vi "LC-MISDK_UserCalibration__.vi"() -> ()   [LabVIEW 2015]
uses:
  C:/Program Files (x86)/National Instruments/LabVIEW 2015/LC-MISDK.dll
  Program Files (x86)/National Instruments/LabVIEW 2015/LC-MISDK.dll
panel:
  in  "タイムスタンプ":timestamp
  out "数値":dbl
  out "error out":errorcluster caption="エラー出力"
  out "ErrorCode":dbl
  in  "Before_B 2":bool
  in  "Before_G 2":bool
  in  "Before_R 2":bool
  in  "Before_W 2":bool
  in  "After_B":T1
  in  "After_G":T2
  in  "After_R":T3
  in  "After_W":T4
  in  "Before_B":T5
  in  "Before_G":T6
  in  "Before_R":T7
  in  "Before_W":T8
  out "Error Message":string
  in  "EXIT":bool
  in  "Calib":bool
  in  "ID":string
  in  "Color Space":T9(ring)
  in  "Calib.Ch":T10(ring)
  in  "Type of Calibration":enum32{"Single-Point", "RGB", "WRGB"}(radio)
  # "Value before Calibration"
  # "Value after Calibration"
  # "Lv"
  # "u"
  # "v"
  # "Lv"
  # "u"
  # "v"
  # "White"
  # "White"
  # "Red"
  # "Red"
  # "Green"
  # "Green"
  # "Blue"
  # "Blue"
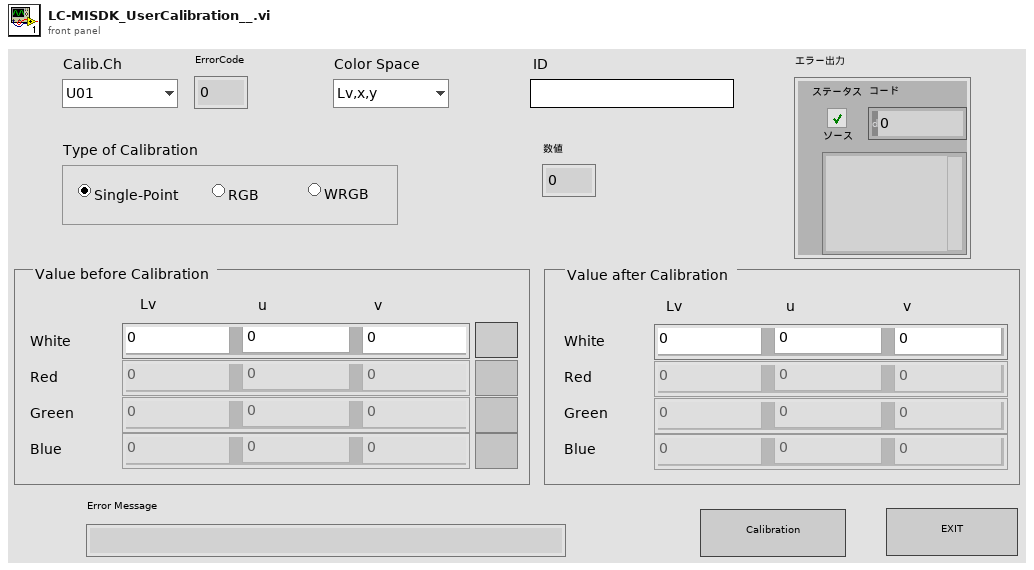
[diagram p1: front panel]
types:
  T1 = cluster{"After_B1":dbl, "After_B2":dbl, "After_B3":dbl}
  T2 = cluster{"After_G1":dbl, "After_G2":dbl, "After_G3":dbl}
  T3 = cluster{"After_R1":dbl, "After_R2":dbl, "After_R3":dbl}
  T4 = cluster{"After_W1":dbl, "After_W2":dbl, "After_W3":dbl}
  T5 = cluster{"before_B1":dbl, "Before_B2":dbl, "Before_B3":dbl}
  T6 = cluster{"before_G1":dbl, "Before_G2":dbl, "Before_G3":dbl}
  T7 = cluster{"before_R1":dbl, "Before_R2":dbl, "Before_R3":dbl}
  T8 = cluster{"before_W1":dbl, "Before_W2":dbl, "Before_W3":dbl}
  T9 = enum16{"Lv,x,y", "Lv,u',v'", "Lv,Tcp,duv", "X,Y,Z", "Lv,λd,Pe"}
  T10 = enum16{"U01", "U02", "U03", "U04", "U05", "U06", "U07", "U08", "U09", "U10"}
  T11 = cluster{"get_Item":dbl, "get_Item":dbl, "get_Item":dbl}
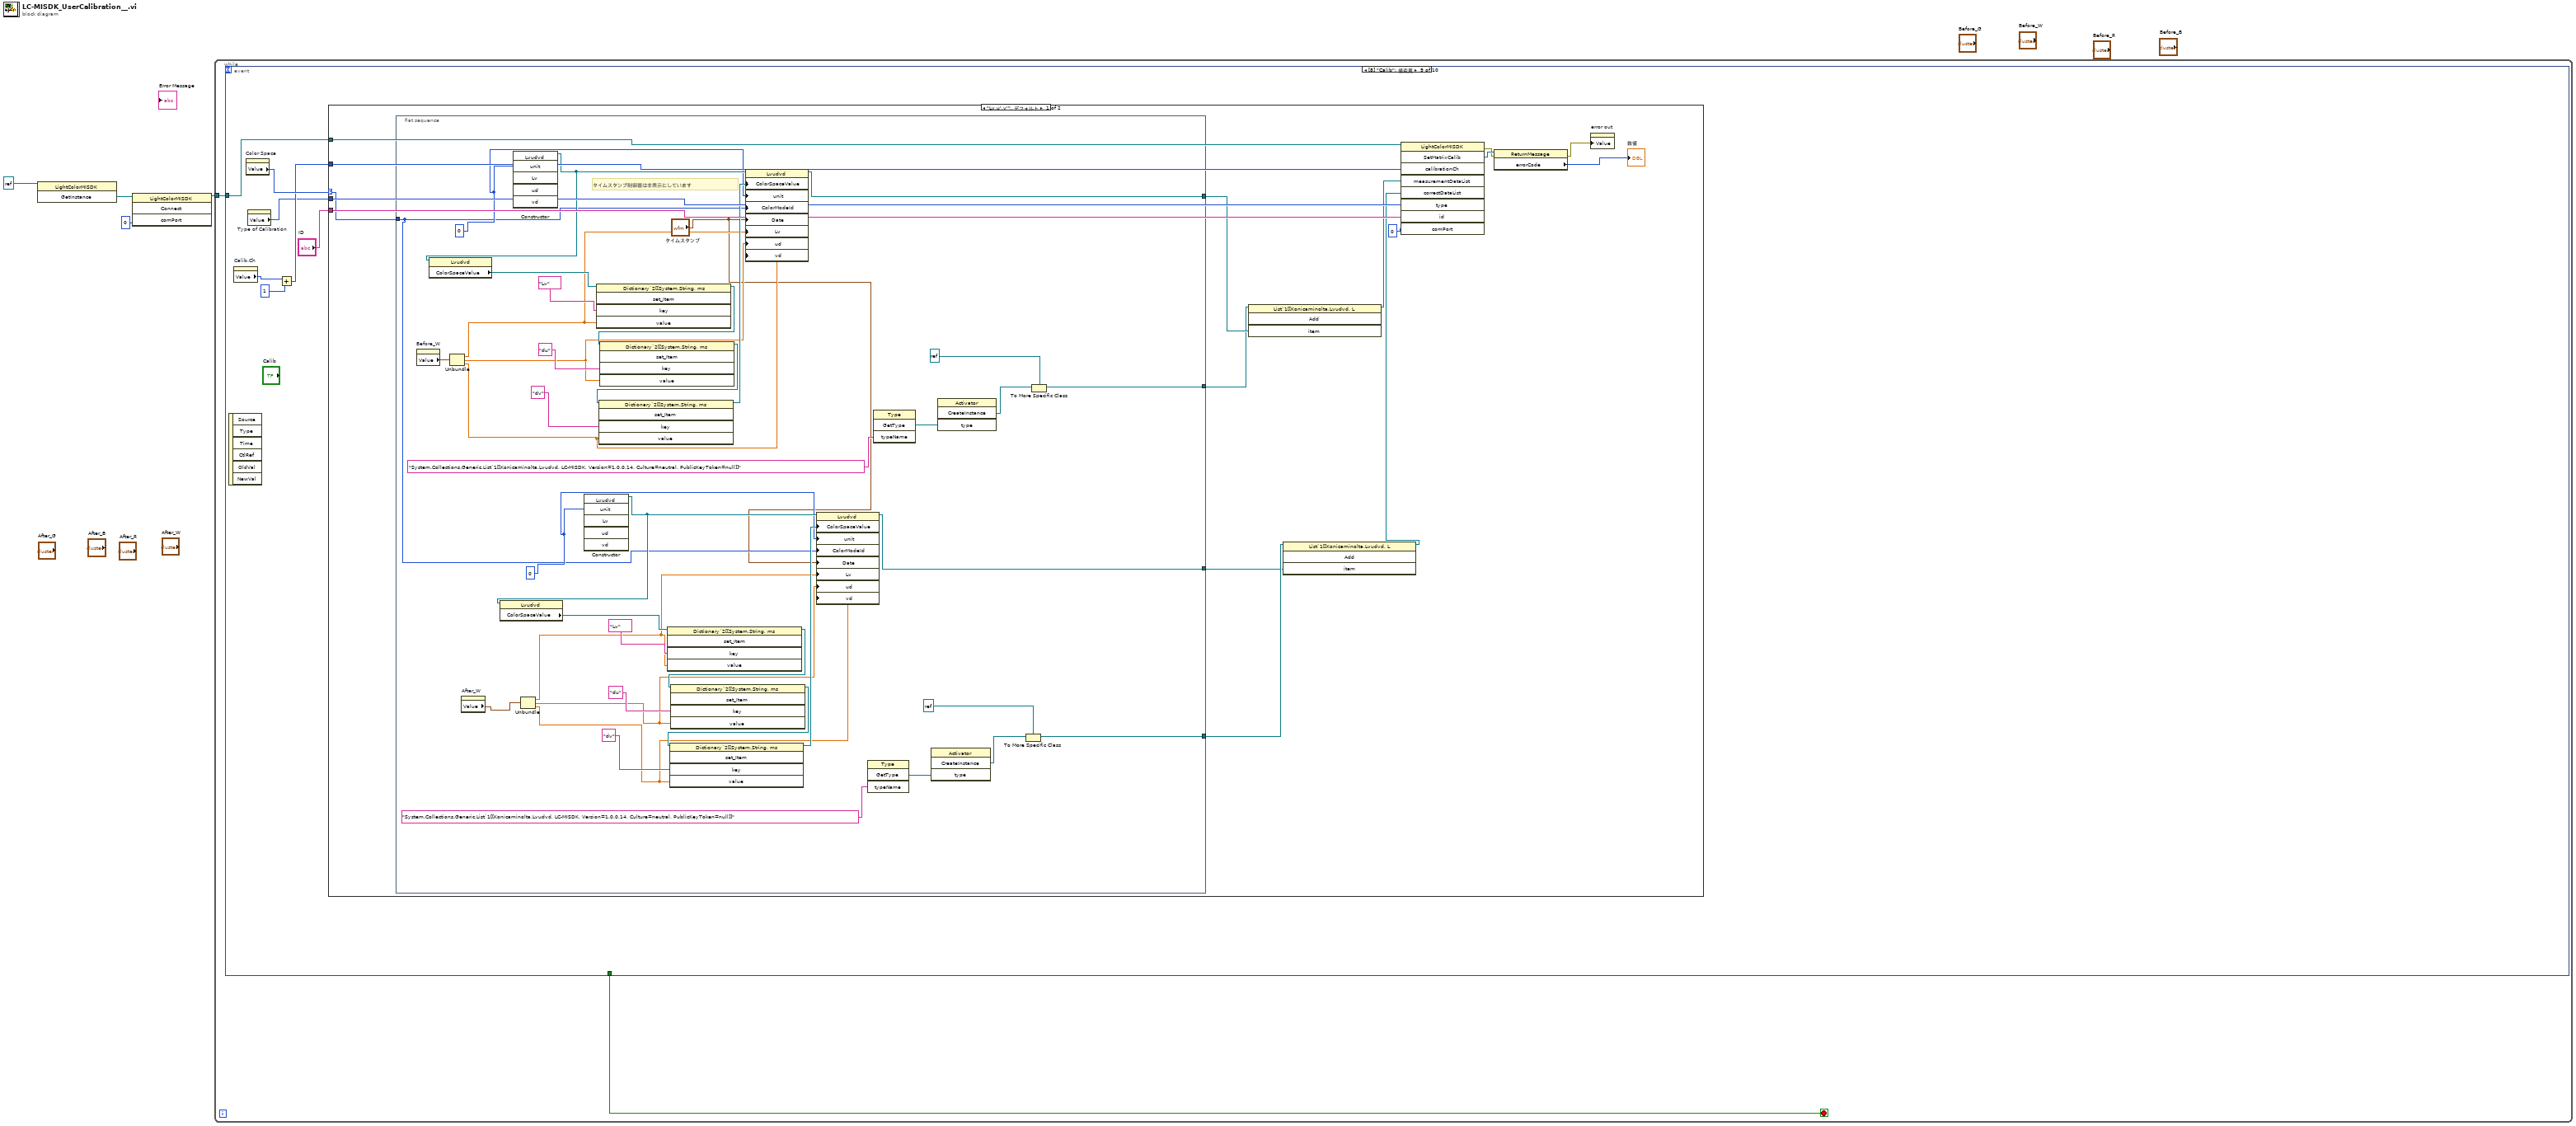
[diagram p0: block diagram]
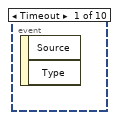
[diagram p2: hidden frame]
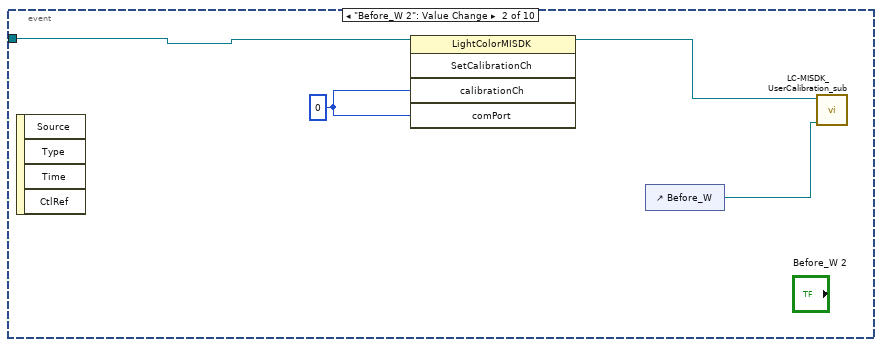
[diagram p3: hidden frame]
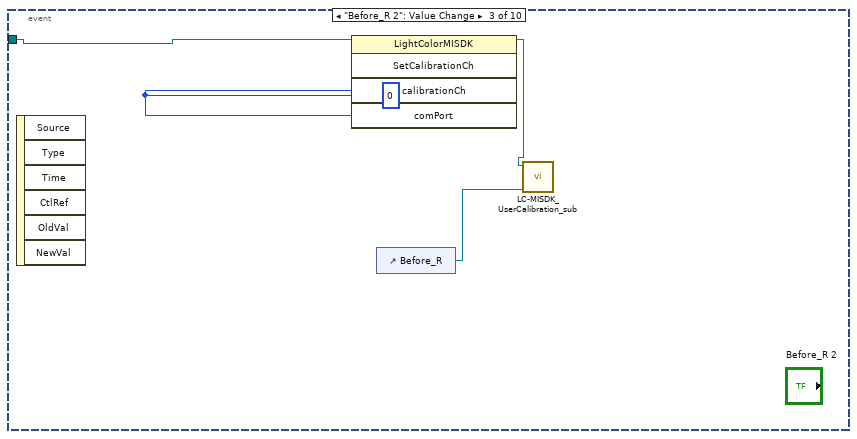
[diagram p4: hidden frame]
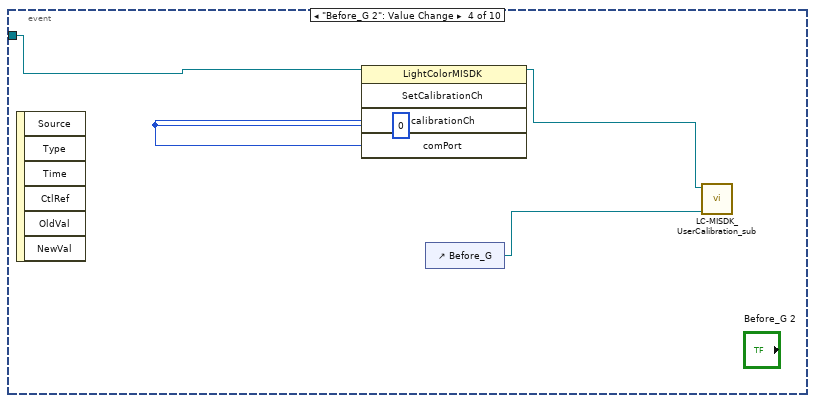
[diagram p5: hidden frame]
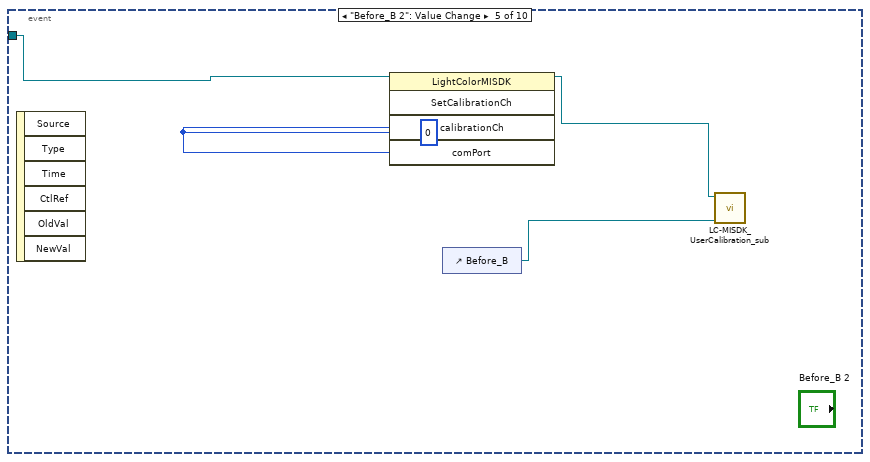
[diagram p6: hidden frame]
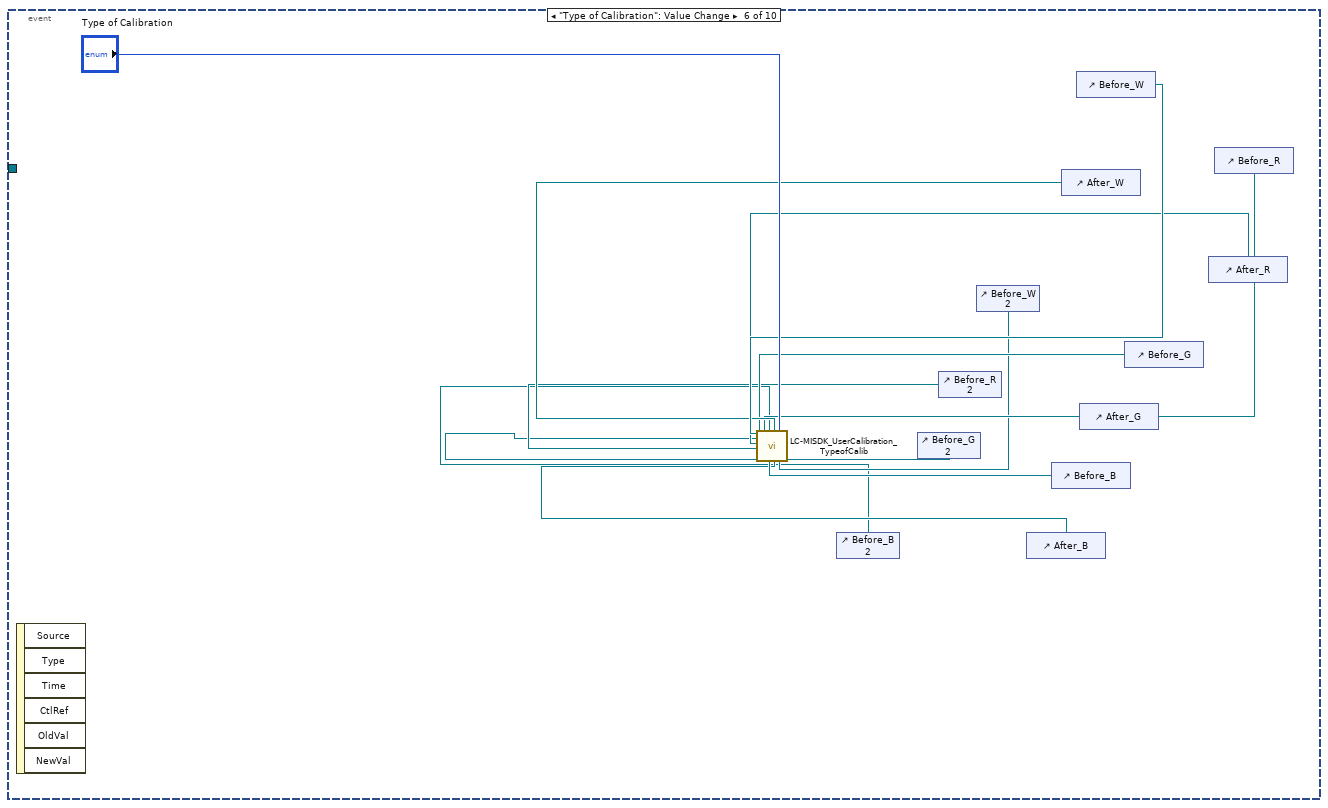
[diagram p7: hidden frame]
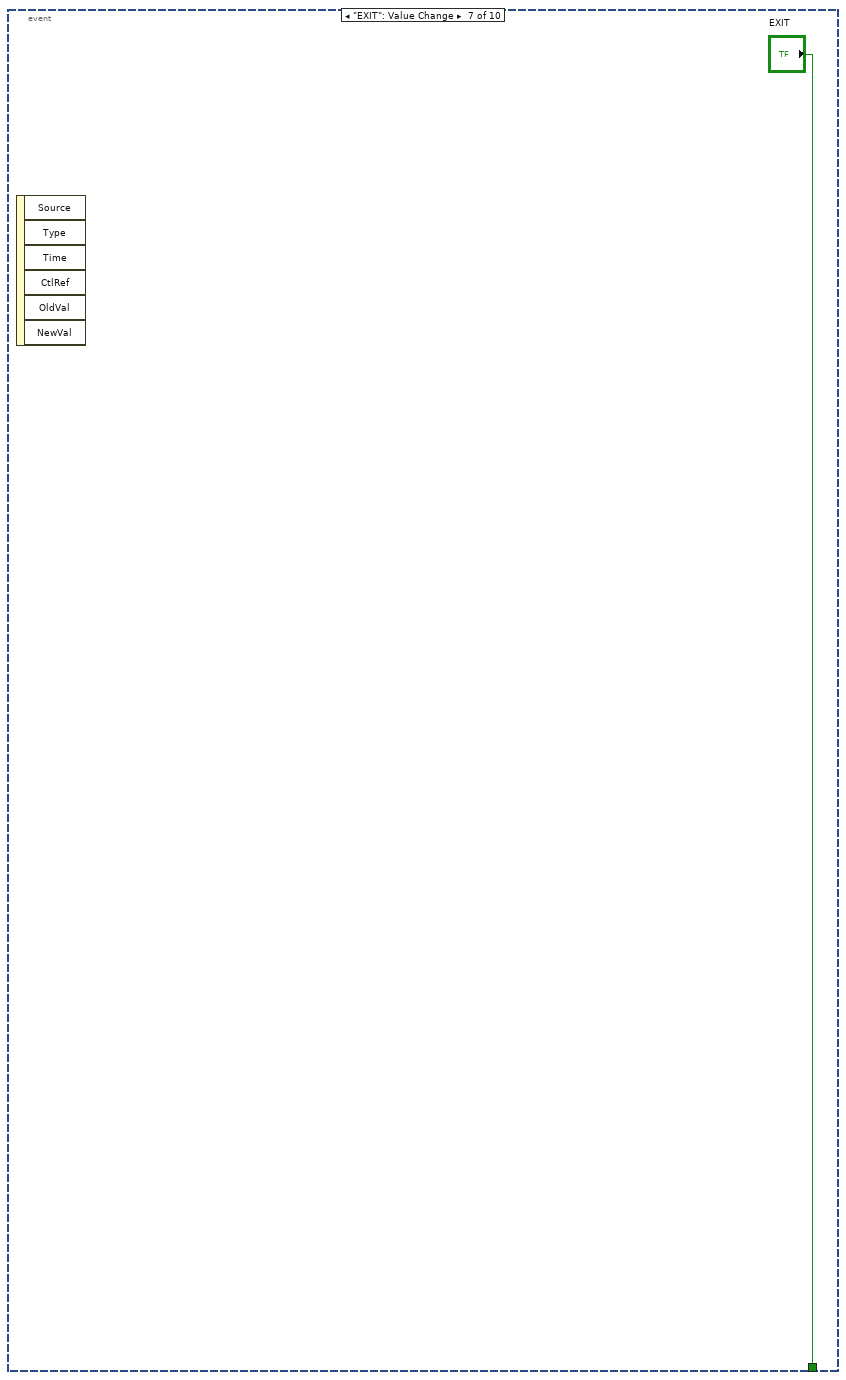
[diagram p8: hidden frame]
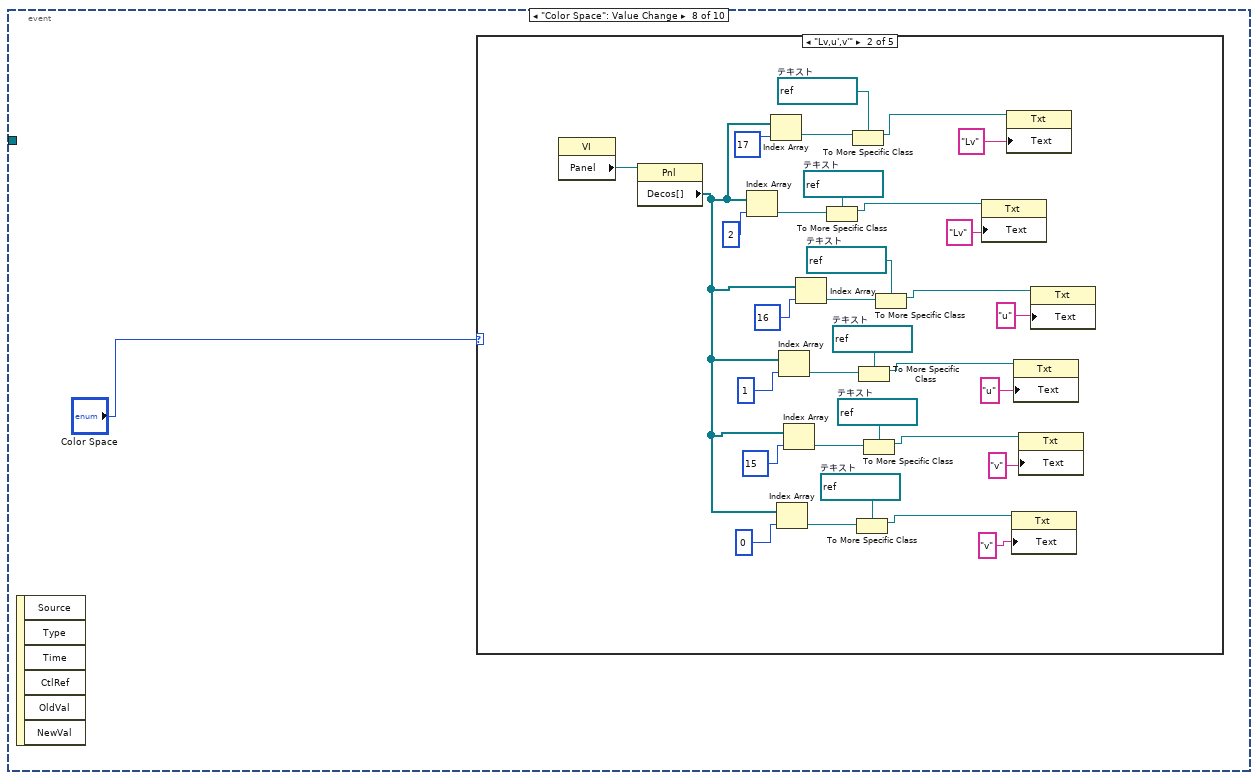
[diagram p9: hidden frame]
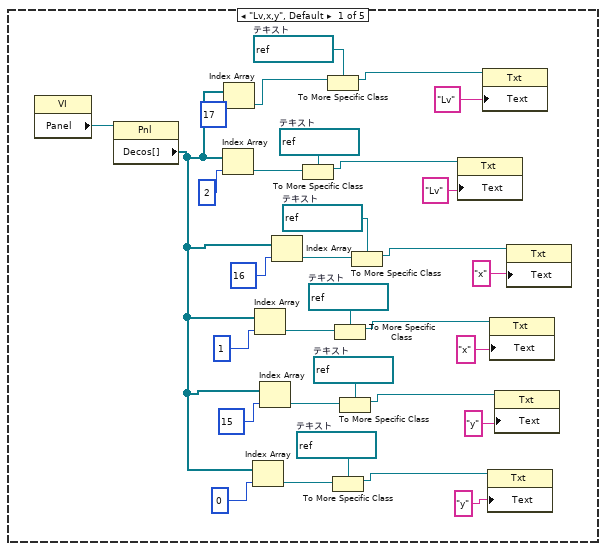
[diagram p10: hidden frame]
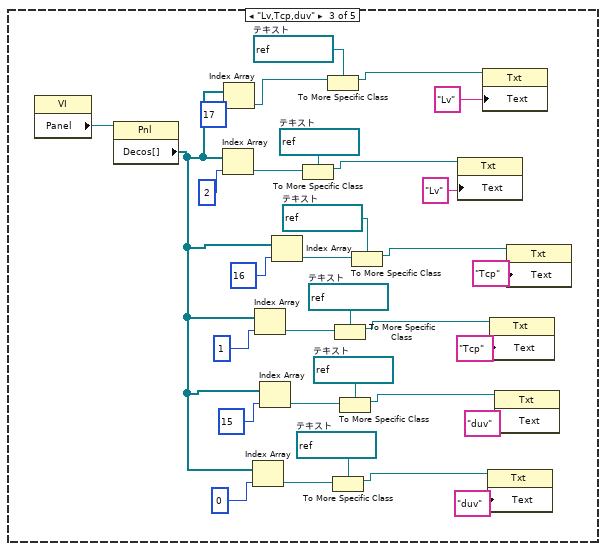
[diagram p11: hidden frame]
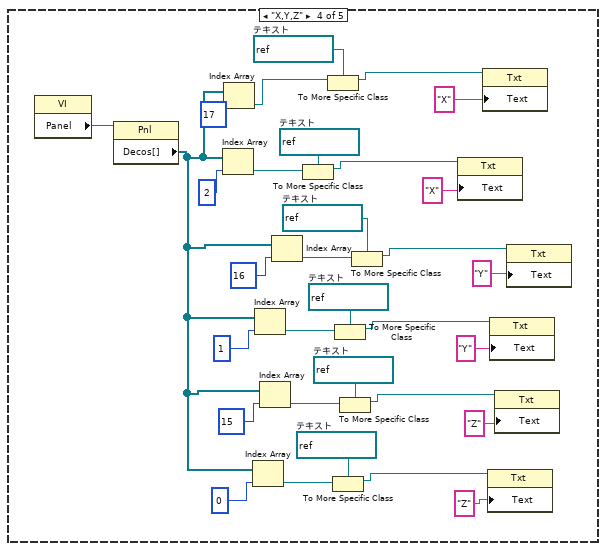
[diagram p12: hidden frame]
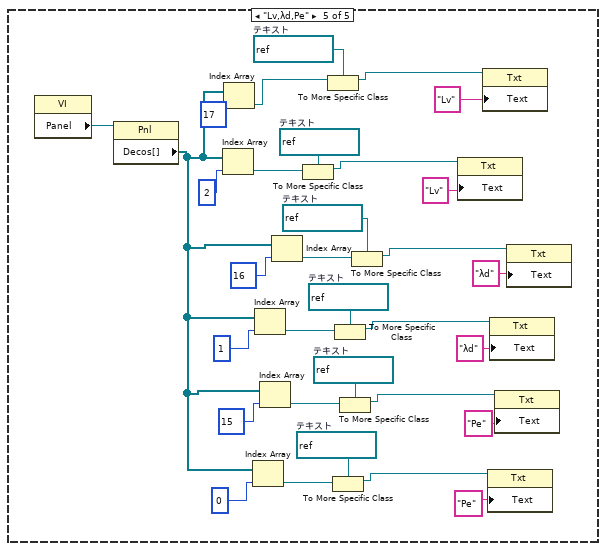
[diagram p13: hidden frame]
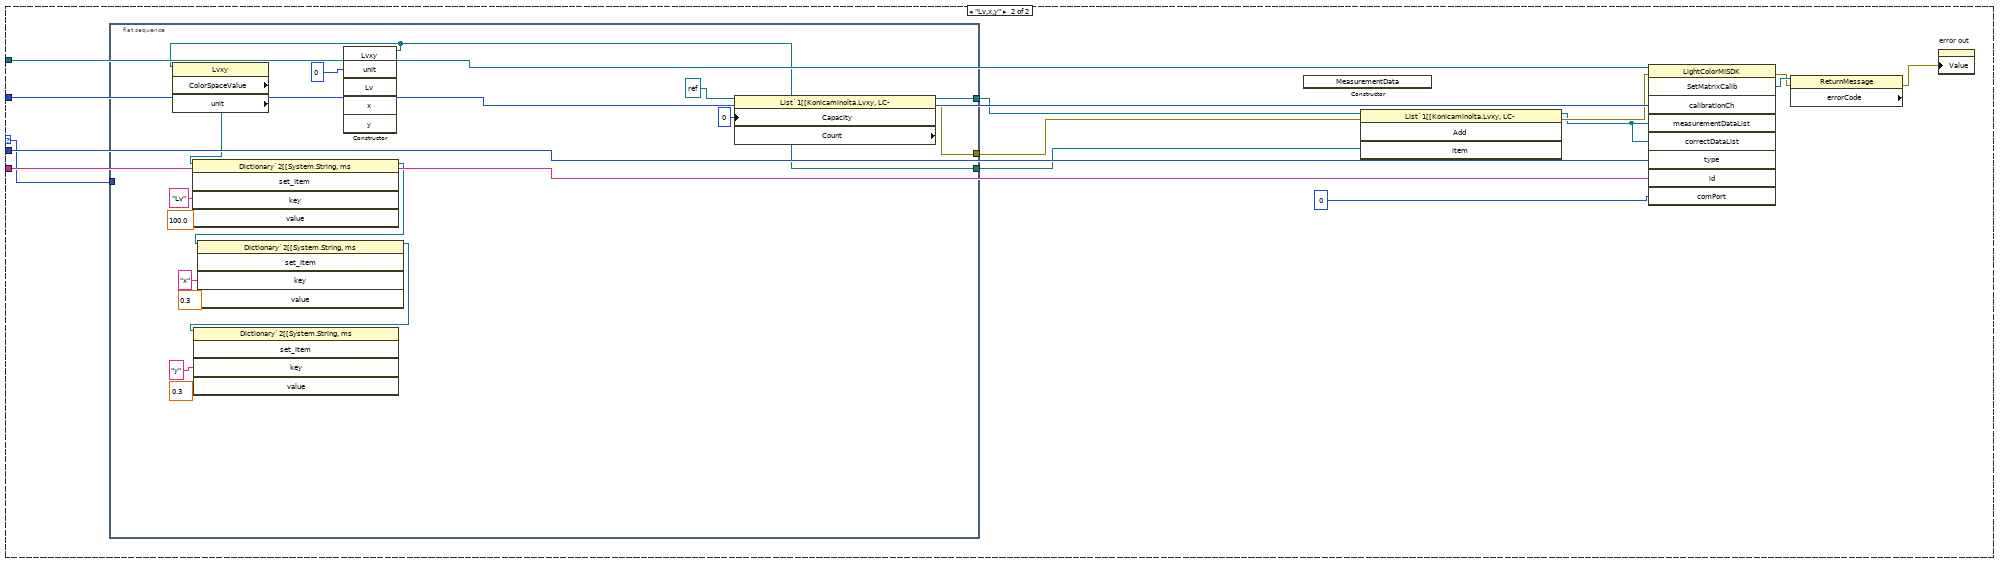
[diagram p14: hidden frame]
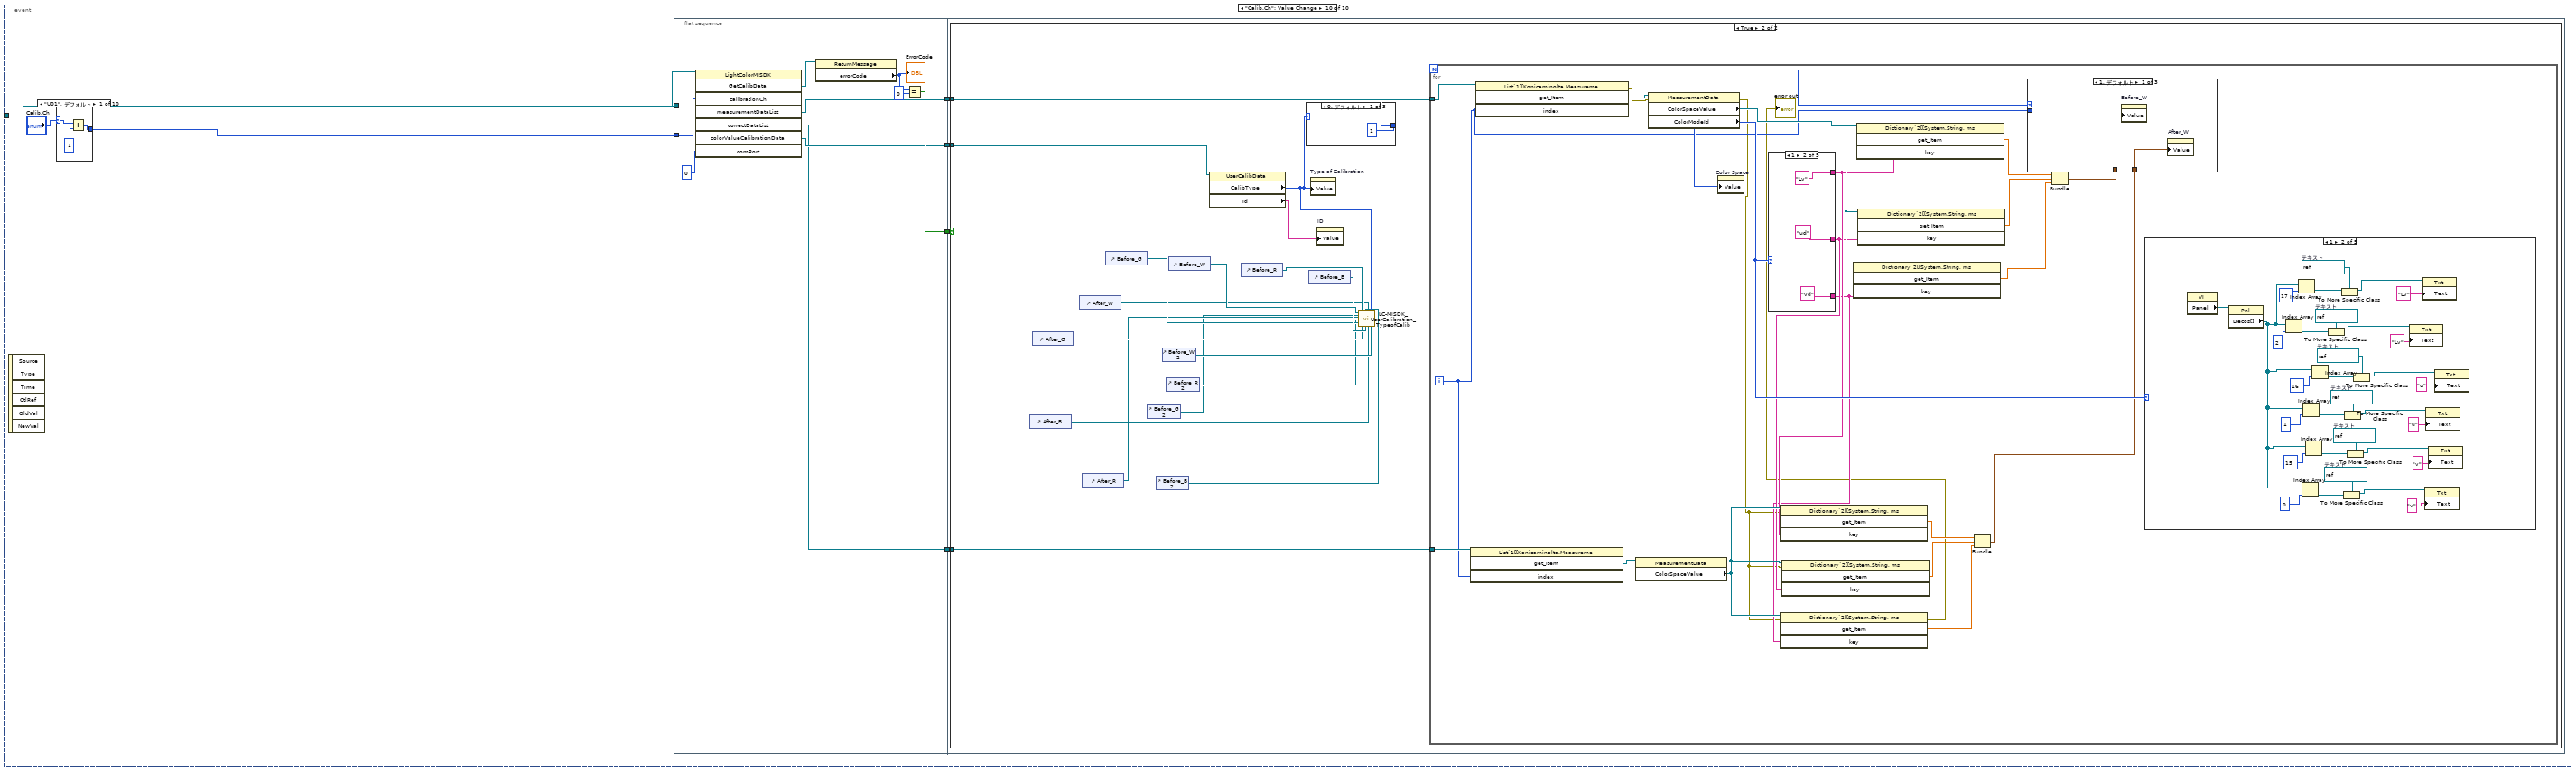
[diagram p15: hidden frame]
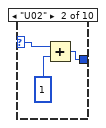
[diagram p16: hidden frame]
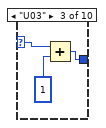
[diagram p17: hidden frame]
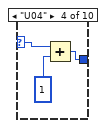
[diagram p18: hidden frame]
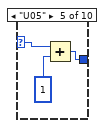
[diagram p19: hidden frame]
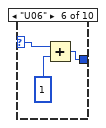
[diagram p20: hidden frame]
diagram:
  n1 = invoke on="インボークノード" class="LightColorMISDK" method="GetInstance"(reference=refnum<k24> refnum ("リファレンス出力")) -> ("GetInstance"=w3:refnum<k24>)  [unwired: 2 in, 2 out]
  n2 = invoke on="インボークノード" class="LightColorMISDK" method="Connect"(reference=w3, "comPort"=0) -> (reference out=w1:refnum<k24>)  [unwired: 2 in, 3 out]
  n3 = while {
    tunnel: w1 -> [w6]
    stop <- w5 stop-if-true
    n4 = event shown="[8] \"Calib\": 値変更" {
      selector: _ -> [_ _ _ _ _ _ _ _ _ _]
      dyn-events: _ -> [_ _ _ _ _ _ _ _ _ _]
      timeout: _ -> [_ _ _ _ _ _ _ _ _ _]
      tunnel: w6 -> [_ w9 w11 w15 w19 _ _ _ w202 w296]
      tunnel: [_ _ _ _ _ _ "EXIT" _ _ _] -> w5
      event Timeout {
        n5 = event-data() -> ()  [unwired: 1 in, 2 out]
      }
      event "Before_W 2": Value Change {
        w7 = 0
        n6 = event-data() -> ()  [unwired: 1 in, 4 out]
        n7 = invoke on="インボークノード" class="LightColorMISDK" method="SetCalibrationCh"(reference=w9, "calibrationCh"=w7, "comPort"=w7) -> (reference out=w8:refnum<k24>)  [unwired: 2 in, 4 out]
        n8 = control-ref of="Before_W"() -> (w10:refnum<vi>)
        n9 = call "LC-MISDK_UserCalibration_sub.vi"(".NET refnum入力"=w8, "Clust refnum"=w10) -> ()  [unwired: 9 in]
      }
      event "Before_R 2": Value Change {
        w13 = 0
        n10 = event-data() -> ()  [unwired: 1 in, 6 out]
        n11 = invoke on="インボークノード" class="LightColorMISDK" method="SetCalibrationCh"(reference=w11, "calibrationCh"=w13, "comPort"=w13) -> (reference out=w12:refnum<k24>)  [unwired: 2 in, 4 out]
        n12 = control-ref of="Before_R"() -> (w14:refnum<vi>)
        n13 = call "LC-MISDK_UserCalibration_sub.vi"(".NET refnum入力"=w12, "Clust refnum"=w14) -> ()  [unwired: 9 in]
      }
      event "Before_G 2": Value Change {
        w17 = 0
        n14 = event-data() -> ()  [unwired: 1 in, 6 out]
        n15 = invoke on="インボークノード" class="LightColorMISDK" method="SetCalibrationCh"(reference=w15, "calibrationCh"=w17, "comPort"=w17) -> (reference out=w16:refnum<k24>)  [unwired: 2 in, 4 out]
        n16 = control-ref of="Before_G"() -> (w18:refnum<vi>)
        n17 = call "LC-MISDK_UserCalibration_sub.vi"(".NET refnum入力"=w16, "Clust refnum"=w18) -> ()  [unwired: 9 in]
      }
      event "Before_B 2": Value Change {
        w21 = 0
        n18 = event-data() -> ()  [unwired: 1 in, 6 out]
        n19 = invoke on="インボークノード" class="LightColorMISDK" method="SetCalibrationCh"(reference=w19, "calibrationCh"=w21, "comPort"=w21) -> (reference out=w20:refnum<k24>)  [unwired: 2 in, 4 out]
        n20 = control-ref of="Before_B"() -> (w22:refnum<vi>)
        n21 = call "LC-MISDK_UserCalibration_sub.vi"(".NET refnum入力"=w20, "Clust refnum"=w22) -> ()  [unwired: 9 in]
      }
      event "Type of Calibration": Value Change {
        n22 = event-data() -> ()  [unwired: 1 in, 6 out]
        n23 = control-ref of="Before_B 2"() -> (w23:refnum<vi>)
        n24 = control-ref of="Before_G 2"() -> (w24:refnum<vi>)
        n25 = control-ref of="Before_R 2"() -> (w25:refnum<vi>)
        n26 = control-ref of="Before_W 2"() -> (w26:refnum<vi>)
        n27 = control-ref of="After_B"() -> (w27:refnum<vi>)
        n28 = control-ref of="Before_B"() -> (w28:refnum<vi>)
        n29 = control-ref of="After_W"() -> (w33:refnum<vi>)
        n30 = control-ref of="Before_W"() -> (w34:refnum<vi>)
        n31 = control-ref of="After_G"() -> (w29:refnum<vi>)
        n32 = control-ref of="Before_G"() -> (w30:refnum<vi>)
        n33 = control-ref of="After_R"() -> (w31:refnum<vi>)
        n34 = control-ref of="Before_R"() -> (w32:refnum<vi>)
        n35 = call "LC-MISDK_UserCalibration_TypeofCalib.vi"("Cluster入力"=w34, "Bool refnum 3"=w24, "Clust refnum 4"=w31, "Bool refnum 2"=w25, "Clust refnum 5"=w30, "Clust refnum 3"=w32, "Clust refnum 6"=w29, "Bool refnum 4"=w23, "Clust refnum 7"=w28, "Clust refnum入力"=w33, "Clust refnum 8"=w27, "Type of Calibration"="Type of Calibration", "Bool refnum"=w26) -> ()  [unwired: 7 in]
      }
      event "EXIT": Value Change {
        n36 = event-data() -> ()  [unwired: 1 in, 6 out]
      }
      event "Color Space": Value Change {
        n37 = event-data() -> ()  [unwired: 1 in, 6 out]
        n38 = case shown="\"Lv,u',v'\"" "Color Space" {
          frame "Lv,x,y", Default {
            w41 = refnum<vi> refnum  # テキスト
            w46 = refnum<vi> refnum  # テキスト
            w49 = refnum<vi> refnum  # テキスト
            w56 = refnum<vi> refnum  # テキスト
            w61 = refnum<vi> refnum  # テキスト
            w66 = refnum<vi> refnum  # テキスト
            n39 = property class="VI"() -> ("Panel"=w69:refnum<vi>)  [unwired: 2 in, 2 out]
            n40 = property class="Pnl"(reference=w69) -> ("Decos[]"=w38:refnum<vi>[])  [unwired: 1 in, 2 out]
            n41 = Index Array(array=w38, index=2) -> (element=w68:refnum<vi>)
            n42 = Index Array(array=w38, index=17) -> (element=w51:refnum<vi>)
            n43 = Index Array(array=w38, index=0) -> (element=w58:refnum<vi>)
            n44 = Index Array(array=w38, index=1) -> (element=w63:refnum<vi>)
            n45 = Index Array(array=w38, index=15) -> (element=w43:refnum<vi>)
            n46 = Index Array(array=w38, index=16) -> (element=w48:refnum<vi>)
            n47 = To More Specific Class(target class=w66, reference=w68) -> (specific class reference=w67:refnum<vi>)  [unwired: 1 in, 1 out]
            n48 = To More Specific Class(target class=w49, reference=w51) -> (specific class reference=w53:refnum<vi>)  [unwired: 1 in, 1 out]
            n49 = To More Specific Class(target class=w56, reference=w58) -> (specific class reference=w57:refnum<vi>)  [unwired: 1 in, 1 out]
            n50 = To More Specific Class(target class=w61, reference=w63) -> (specific class reference=w62:refnum<vi>)  [unwired: 1 in, 1 out]
            n51 = To More Specific Class(target class=w41, reference=w43) -> (specific class reference=w42:refnum<vi>)  [unwired: 1 in, 1 out]
            n52 = To More Specific Class(target class=w46, reference=w48) -> (specific class reference=w47:refnum<vi>)  [unwired: 1 in, 1 out]
            n53 = property class="Txt"(reference=w67, "Text"="Lv") -> ()  [unwired: 1 in, 2 out]
            n54 = property class="Txt"(reference=w53, "Text"="Lv") -> ()  [unwired: 1 in, 2 out]
            n55 = property class="Txt"(reference=w57, "Text"="y") -> ()  [unwired: 1 in, 2 out]
            n56 = property class="Txt"(reference=w62, "Text"="x") -> ()  [unwired: 1 in, 2 out]
            n57 = property class="Txt"(reference=w42, "Text"="y") -> ()  [unwired: 1 in, 2 out]
            n58 = property class="Txt"(reference=w47, "Text"="x") -> ()  [unwired: 1 in, 2 out]
          }
          frame "Lv,u',v'" {
            w73 = refnum<vi> refnum  # テキスト
            w78 = refnum<vi> refnum  # テキスト
            w81 = refnum<vi> refnum  # テキスト
            w88 = refnum<vi> refnum  # テキスト
            w93 = refnum<vi> refnum  # テキスト
            w98 = refnum<vi> refnum  # テキスト
            n59 = property class="VI"() -> ("Panel"=w101:refnum<vi>)  [unwired: 2 in, 2 out]
            n60 = property class="Pnl"(reference=w101) -> ("Decos[]"=w70:refnum<vi>[])  [unwired: 1 in, 2 out]
            n61 = Index Array(array=w70, index=2) -> (element=w100:refnum<vi>)
            n62 = Index Array(array=w70, index=17) -> (element=w83:refnum<vi>)
            n63 = Index Array(array=w70, index=0) -> (element=w90:refnum<vi>)
            n64 = Index Array(array=w70, index=1) -> (element=w95:refnum<vi>)
            n65 = Index Array(array=w70, index=15) -> (element=w75:refnum<vi>)
            n66 = Index Array(array=w70, index=16) -> (element=w80:refnum<vi>)
            n67 = To More Specific Class(target class=w98, reference=w100) -> (specific class reference=w99:refnum<vi>)  [unwired: 1 in, 1 out]
            n68 = To More Specific Class(target class=w81, reference=w83) -> (specific class reference=w85:refnum<vi>)  [unwired: 1 in, 1 out]
            n69 = To More Specific Class(target class=w88, reference=w90) -> (specific class reference=w89:refnum<vi>)  [unwired: 1 in, 1 out]
            n70 = To More Specific Class(target class=w93, reference=w95) -> (specific class reference=w94:refnum<vi>)  [unwired: 1 in, 1 out]
            n71 = To More Specific Class(target class=w73, reference=w75) -> (specific class reference=w74:refnum<vi>)  [unwired: 1 in, 1 out]
            n72 = To More Specific Class(target class=w78, reference=w80) -> (specific class reference=w79:refnum<vi>)  [unwired: 1 in, 1 out]
            n73 = property class="Txt"(reference=w99, "Text"="Lv") -> ()  [unwired: 1 in, 2 out]
            n74 = property class="Txt"(reference=w85, "Text"="Lv") -> ()  [unwired: 1 in, 2 out]
            n75 = property class="Txt"(reference=w89, "Text"="v") -> ()  [unwired: 1 in, 2 out]
            n76 = property class="Txt"(reference=w94, "Text"="u") -> ()  [unwired: 1 in, 2 out]
            n77 = property class="Txt"(reference=w74, "Text"="v") -> ()  [unwired: 1 in, 2 out]
            n78 = property class="Txt"(reference=w79, "Text"="u") -> ()  [unwired: 1 in, 2 out]
          }
          frame "Lv,Tcp,duv" {
            w105 = refnum<vi> refnum  # テキスト
            w110 = refnum<vi> refnum  # テキスト
            w113 = refnum<vi> refnum  # テキスト
            w120 = refnum<vi> refnum  # テキスト
            w125 = refnum<vi> refnum  # テキスト
            w130 = refnum<vi> refnum  # テキスト
            n79 = property class="VI"() -> ("Panel"=w133:refnum<vi>)  [unwired: 2 in, 2 out]
            n80 = property class="Pnl"(reference=w133) -> ("Decos[]"=w102:refnum<vi>[])  [unwired: 1 in, 2 out]
            n81 = Index Array(array=w102, index=2) -> (element=w132:refnum<vi>)
            n82 = Index Array(array=w102, index=17) -> (element=w115:refnum<vi>)
            n83 = Index Array(array=w102, index=0) -> (element=w122:refnum<vi>)
            n84 = Index Array(array=w102, index=1) -> (element=w127:refnum<vi>)
            n85 = Index Array(array=w102, index=15) -> (element=w107:refnum<vi>)
            n86 = Index Array(array=w102, index=16) -> (element=w112:refnum<vi>)
            n87 = To More Specific Class(target class=w130, reference=w132) -> (specific class reference=w131:refnum<vi>)  [unwired: 1 in, 1 out]
            n88 = To More Specific Class(target class=w113, reference=w115) -> (specific class reference=w117:refnum<vi>)  [unwired: 1 in, 1 out]
            n89 = To More Specific Class(target class=w120, reference=w122) -> (specific class reference=w121:refnum<vi>)  [unwired: 1 in, 1 out]
            n90 = To More Specific Class(target class=w125, reference=w127) -> (specific class reference=w126:refnum<vi>)  [unwired: 1 in, 1 out]
            n91 = To More Specific Class(target class=w105, reference=w107) -> (specific class reference=w106:refnum<vi>)  [unwired: 1 in, 1 out]
            n92 = To More Specific Class(target class=w110, reference=w112) -> (specific class reference=w111:refnum<vi>)  [unwired: 1 in, 1 out]
            n93 = property class="Txt"(reference=w131, "Text"="Lv") -> ()  [unwired: 1 in, 2 out]
            n94 = property class="Txt"(reference=w117, "Text"="Lv") -> ()  [unwired: 1 in, 2 out]
            n95 = property class="Txt"(reference=w121, "Text"="duv") -> ()  [unwired: 1 in, 2 out]
            n96 = property class="Txt"(reference=w126, "Text"="Tcp") -> ()  [unwired: 1 in, 2 out]
            n97 = property class="Txt"(reference=w106, "Text"="duv") -> ()  [unwired: 1 in, 2 out]
            n98 = property class="Txt"(reference=w111, "Text"="Tcp") -> ()  [unwired: 1 in, 2 out]
          }
          frame "X,Y,Z" {
            w137 = refnum<vi> refnum  # テキスト
            w142 = refnum<vi> refnum  # テキスト
            w145 = refnum<vi> refnum  # テキスト
            w152 = refnum<vi> refnum  # テキスト
            w157 = refnum<vi> refnum  # テキスト
            w162 = refnum<vi> refnum  # テキスト
            n99 = property class="VI"() -> ("Panel"=w165:refnum<vi>)  [unwired: 2 in, 2 out]
            n100 = property class="Pnl"(reference=w165) -> ("Decos[]"=w134:refnum<vi>[])  [unwired: 1 in, 2 out]
            n101 = Index Array(array=w134, index=2) -> (element=w164:refnum<vi>)
            n102 = Index Array(array=w134, index=17) -> (element=w147:refnum<vi>)
            n103 = Index Array(array=w134, index=0) -> (element=w154:refnum<vi>)
            n104 = Index Array(array=w134, index=1) -> (element=w159:refnum<vi>)
            n105 = Index Array(array=w134, index=15) -> (element=w139:refnum<vi>)
            n106 = Index Array(array=w134, index=16) -> (element=w144:refnum<vi>)
            n107 = To More Specific Class(target class=w162, reference=w164) -> (specific class reference=w163:refnum<vi>)  [unwired: 1 in, 1 out]
            n108 = To More Specific Class(target class=w145, reference=w147) -> (specific class reference=w149:refnum<vi>)  [unwired: 1 in, 1 out]
            n109 = To More Specific Class(target class=w152, reference=w154) -> (specific class reference=w153:refnum<vi>)  [unwired: 1 in, 1 out]
            n110 = To More Specific Class(target class=w157, reference=w159) -> (specific class reference=w158:refnum<vi>)  [unwired: 1 in, 1 out]
            n111 = To More Specific Class(target class=w137, reference=w139) -> (specific class reference=w138:refnum<vi>)  [unwired: 1 in, 1 out]
            n112 = To More Specific Class(target class=w142, reference=w144) -> (specific class reference=w143:refnum<vi>)  [unwired: 1 in, 1 out]
            n113 = property class="Txt"(reference=w163, "Text"="X") -> ()  [unwired: 1 in, 2 out]
            n114 = property class="Txt"(reference=w149, "Text"="X") -> ()  [unwired: 1 in, 2 out]
            n115 = property class="Txt"(reference=w153, "Text"="Z") -> ()  [unwired: 1 in, 2 out]
            n116 = property class="Txt"(reference=w158, "Text"="Y") -> ()  [unwired: 1 in, 2 out]
            n117 = property class="Txt"(reference=w138, "Text"="Z") -> ()  [unwired: 1 in, 2 out]
            n118 = property class="Txt"(reference=w143, "Text"="Y") -> ()  [unwired: 1 in, 2 out]
          }
          frame "Lv,λd,Pe" {
            w169 = refnum<vi> refnum  # テキスト
            w174 = refnum<vi> refnum  # テキスト
            w177 = refnum<vi> refnum  # テキスト
            w184 = refnum<vi> refnum  # テキスト
            w189 = refnum<vi> refnum  # テキスト
            w194 = refnum<vi> refnum  # テキスト
            n119 = property class="VI"() -> ("Panel"=w197:refnum<vi>)  [unwired: 2 in, 2 out]
            n120 = property class="Pnl"(reference=w197) -> ("Decos[]"=w166:refnum<vi>[])  [unwired: 1 in, 2 out]
            n121 = Index Array(array=w166, index=2) -> (element=w196:refnum<vi>)
            n122 = Index Array(array=w166, index=17) -> (element=w179:refnum<vi>)
            n123 = Index Array(array=w166, index=0) -> (element=w186:refnum<vi>)
            n124 = Index Array(array=w166, index=1) -> (element=w191:refnum<vi>)
            n125 = Index Array(array=w166, index=15) -> (element=w171:refnum<vi>)
            n126 = Index Array(array=w166, index=16) -> (element=w176:refnum<vi>)
            n127 = To More Specific Class(target class=w194, reference=w196) -> (specific class reference=w195:refnum<vi>)  [unwired: 1 in, 1 out]
            n128 = To More Specific Class(target class=w177, reference=w179) -> (specific class reference=w181:refnum<vi>)  [unwired: 1 in, 1 out]
            n129 = To More Specific Class(target class=w184, reference=w186) -> (specific class reference=w185:refnum<vi>)  [unwired: 1 in, 1 out]
            n130 = To More Specific Class(target class=w189, reference=w191) -> (specific class reference=w190:refnum<vi>)  [unwired: 1 in, 1 out]
            n131 = To More Specific Class(target class=w169, reference=w171) -> (specific class reference=w170:refnum<vi>)  [unwired: 1 in, 1 out]
            n132 = To More Specific Class(target class=w174, reference=w176) -> (specific class reference=w175:refnum<vi>)  [unwired: 1 in, 1 out]
            n133 = property class="Txt"(reference=w195, "Text"="Lv") -> ()  [unwired: 1 in, 2 out]
            n134 = property class="Txt"(reference=w181, "Text"="Lv") -> ()  [unwired: 1 in, 2 out]
            n135 = property class="Txt"(reference=w185, "Text"="Pe") -> ()  [unwired: 1 in, 2 out]
            n136 = property class="Txt"(reference=w190, "Text"="λd") -> ()  [unwired: 1 in, 2 out]
            n137 = property class="Txt"(reference=w170, "Text"="Pe") -> ()  [unwired: 1 in, 2 out]
            n138 = property class="Txt"(reference=w175, "Text"="λd") -> ()  [unwired: 1 in, 2 out]
          }
        }
      }
      event "Calib": Value Change {
        n139 = event-data() -> ()  [unwired: 1 in, 6 out]
        n140 = property on="Calib.Ch" class="Enum （指定）"() -> ("Value"=w201:T10)  [unwired: 2 in, 2 out]
        n141 = property on="Color Space" class="Enum （指定）"() -> ("Value"=w203:T9)  [unwired: 2 in, 2 out]
        n142 = property on="Type of Calibration" class="RadioBtnsControl （指定）"() -> ("Value"=w199:enum32{"Single-Point", "RGB", "WRGB"})  [unwired: 2 in, 2 out]
        n143 = Add(x=w201, y=1) -> (x+y=w200:i32)
        n144 = case shown="\"Lv,u',v'\", デフォルト" w203 {
          selector: w203 -> [w212 w267]
          tunnel: w202 -> [w220 w274]
          tunnel: w200 -> [w219 w273]
          tunnel: "ID" -> [w218 w272]
          tunnel: w199 -> [w217 w271]
          frame "Lv,u',v'", Default {
            n145 = flat-sequence {
              tunnel: [w251] -> w210
              tunnel: w212 -> [w231]
              tunnel: [w247] -> w209
              tunnel: [w227] -> w207
              tunnel: [w226] -> w206
              frame #0 {
                w237 = 0
                w253 = 0
                # "タイムスタンプ制御器は非表示にしています"
                n146 = property on="Before_W" class="Clust （指定）"() -> ("Value"=w245:T8)  [unwired: 2 in, 2 out]
                n147 = Unbundle(w245) -> ("before_W1"=w224:dbl, "Before_W2"=w223:dbl, "Before_W3"=w222:dbl)
                n148 = property on="After_W" class="Clust （指定）"() -> ("Value"=w232:T4)  [unwired: 2 in, 2 out]
                n149 = constructor class="Lvudvd"("unit"=w253) -> (reference out=w254:refnum<k24>)  [unwired: 6 in, 6 out]
                n150 = property class="Lvudvd"(reference=w254) -> ("ColorSpaceValue"=w252:refnum<k24>)  [unwired: 1 in, 2 out]
                n151 = Unbundle(w232) -> ("After_W1"=w235:dbl, "After_W2"=w234:dbl, "After_W3"=w233:dbl)
                n152 = constructor class="Lvudvd"("unit"=w237) -> (reference out=w238:refnum<k24>)  [unwired: 6 in, 6 out]
                n153 = property class="Lvudvd"(reference=w238) -> ("ColorSpaceValue"=w236:refnum<k24>)  [unwired: 1 in, 2 out]
                n154 = invoke on="インボークノード" class="Dictionary`2[[System.String, ms" method="set_Item"(reference=w252, "key"="Lv", "value"=w224) -> (reference out=w258:refnum<k24>)  [unwired: 2 in, 4 out]
                n155 = invoke class="Dictionary`2[[System.String, ms" method="set_Item"(reference=w258, "key"="du", "value"=w223) -> (reference out=w257:refnum<k24>)  [unwired: 2 in, 4 out]
                n156 = invoke class="Dictionary`2[[System.String, ms" method="set_Item"(reference=w257, "key"="dv", "value"=w222) -> (reference out=w255:refnum<k24>)  [unwired: 2 in, 4 out]
                n157 = invoke on="インボークノード" class="Dictionary`2[[System.String, ms" method="set_Item"(reference=w236, "key"="Lv", "value"=w235) -> (reference out=w242:refnum<k24>)  [unwired: 2 in, 4 out]
                n158 = invoke class="Dictionary`2[[System.String, ms" method="set_Item"(reference=w242, "key"="du", "value"=w234) -> (reference out=w241:refnum<k24>)  [unwired: 2 in, 4 out]
                n159 = invoke class="Dictionary`2[[System.String, ms" method="set_Item"(reference=w241, "key"="dv", "value"=w233) -> (reference out=w239:refnum<k24>)  [unwired: 2 in, 4 out]
                n160 = property class="Lvudvd"(reference=w254, "ColorSpaceValue"=w255, "unit"=w253, "ColorModeId"=w231, "Date"="タイムスタンプ", "Lv"=w224, "ud"=w223, "vd"=w222) -> (reference out=w251:refnum<k24>)  [unwired: 1 in, 1 out]
                n161 = property class="Lvudvd"(reference=w238, "ColorSpaceValue"=w239, "unit"=w237, "ColorModeId"=w231, "Date"="タイムスタンプ", "Lv"=w235, "ud"=w234, "vd"=w233) -> (reference out=w226:refnum<k24>)  [unwired: 1 in, 1 out]
                n162 = invoke on="インボークノード" class="Type" method="GetType"("typeName"="System.Collections.Generic.List`1[[Konicaminolta.Lvudvd, LC-MISDK, Version=1.0.0.14, Culture=neutral, PublicKeyToken=null]]") -> ("GetType"=w230:refnum<k24>)  [unwired: 3 in, 3 out]
                n163 = invoke on="インボークノード" class="Type" method="GetType"("typeName"="System.Collections.Generic.List`1[[Konicaminolta.Lvudvd, LC-MISDK, Version=1.0.0.14, Culture=neutral, PublicKeyToken=null]]") -> ("GetType"=w249:refnum<k24>)  [unwired: 3 in, 3 out]
                n164 = invoke on="インボークノード" class="Activator" method="CreateInstance"("type"=w230) -> ("CreateInstance"=w228:refnum<k24>)  [unwired: 3 in, 3 out]
                n165 = invoke on="インボークノード" class="Activator" method="CreateInstance"("type"=w249) -> ("CreateInstance"=w246:refnum<k24>)  [unwired: 3 in, 3 out]
                n166 = To More Specific Class(target class=refnum<k24> refnum ("リファレンス出力"), reference=w228) -> (specific class reference=w227:refnum<k24>)  [unwired: 1 in, 1 out]
                n167 = To More Specific Class(target class=refnum<k24> refnum ("リファレンス出力"), reference=w246) -> (specific class reference=w247:refnum<k24>)  [unwired: 1 in, 1 out]
              }
            }
            n168 = invoke on="インボークノード" class="List`1[[Konicaminolta.Lvudvd, L" method="Add"(reference=w209, "item"=w210) -> (reference out=w208:refnum<k24>)  [unwired: 2 in, 3 out]
            n169 = invoke on="インボークノード" class="List`1[[Konicaminolta.Lvudvd, L" method="Add"(reference=w207, "item"=w206) -> (reference out=w205:refnum<k24>)  [unwired: 2 in, 3 out]
            n170 = invoke on="インボークノード" class="LightColorMISDK" method="SetMatrixCalib"(reference=w220, "calibrationCh"=w219, "measurementDataList"=w208, "correctDataList"=w205, "type"=w217, "id"=w218, "comPort"=0) -> (error out=w215:errorcluster, "SetMatrixCalib"=w216:refnum<k24>)  [unwired: 2 in, 7 out]
            n171 = property on="プロパティノード" class="ReturnMessage"(reference=w216, error in=w215) -> (error out=w214:errorcluster, "errorCode"=→"数値":i32)  [unwired: 1 out]
            n172 = property on="error out" class="Clust （指定）"("Value"=w214) -> ()  [unwired: 2 in, 2 out]
          }
          frame "Lv,x,y" {
            n173 = flat-sequence {
              tunnel: w267 -> [_]
              tunnel: [w276] -> w265
              tunnel: [w279] -> w262
              tunnel: [w278] -> w261
              frame #0 {
                n174 = constructor class="Lvxy"("unit"=0) -> (reference out=w279:refnum<k24>)  [unwired: 6 in, 6 out]
                n175 = property on="プロパティノード" class="Lvxy" props=["ColorSpaceValue", "unit"](reference=w279) -> ("ColorSpaceValue"=w280:refnum<k24>)  [unwired: 1 in, 3 out]
                n176 = invoke on="インボークノード" class="Dictionary`2[[System.String, ms" method="set_Item"(reference=w280, "key"="Lv", "value"=100.0) -> (reference out=w283:refnum<k24>)  [unwired: 2 in, 4 out]
                n177 = invoke on="インボークノード" class="Dictionary`2[[System.String, ms" method="set_Item"(reference=w283, "key"="x", "value"=0.3) -> (reference out=w282:refnum<k24>)  [unwired: 2 in, 4 out]
                n178 = invoke on="インボークノード" class="Dictionary`2[[System.String, ms" method="set_Item"(reference=w282, "key"="y", "value"=0.3) -> ()  [unwired: 2 in, 5 out]
                n179 = property class="List`1[[Konicaminolta.Lvxy, LC-" props=["Capacity", "Count"](reference=refnum<k24> refnum ("リファレンス出力"), "Capacity"=0) -> (reference out=w278:refnum<k24>, error out=w276:errorcluster)  [unwired: 1 in, 1 out]
              }
            }
            n180 = constructor class="MeasurementData"() -> ()  [unwired: 3 in, 3 out]
            n181 = invoke on="インボークノード" class="List`1[[Konicaminolta.Lvxy, LC-" method="Add"(reference=w261, error in=w265, "item"=w262) -> (reference out=w263:refnum<k24>, error out=w266:errorcluster)  [unwired: 1 in, 2 out]
            n182 = invoke on="インボークノード" class="LightColorMISDK" method="SetMatrixCalib"(reference=w274, error in=w266, "calibrationCh"=w273, "measurementDataList"=w263, "correctDataList"=w263, "type"=w271, "id"=w272, "comPort"=0) -> (error out=w269:errorcluster, "SetMatrixCalib"=w270:refnum<k24>)  [unwired: 1 in, 7 out]
            n183 = property on="プロパティノード" class="ReturnMessage" props=["errorCode"](reference=w270, error in=w269) -> (error out=w268:errorcluster)  [unwired: 2 out]
            n184 = property on="error out" class="Clust （指定）"("Value"=w268) -> ()  [unwired: 2 in, 2 out]
          }
        }
      }
      event "Calib.Ch": Value Change {
        n185 = event-data() -> ()  [unwired: 1 in, 6 out]
        n186 = case shown="\"U01\", デフォルト" "Calib.Ch" {
          selector: "Calib.Ch" -> [w299 w302 w305 w308 w311 w314 w317 w320 w323 w326]
          tunnel: [w297 w300 w303 w306 w309 w312 w315 w318 w321 w324] -> w293
          frame "U01", Default {
            n187 = Add(x=w299, y=1) -> (x+y=w297:i32)
          }
          frame "U02" {
            n188 = Add(x=w302, y=1) -> (x+y=w300:i32)
          }
          frame "U03" {
            n189 = Add(x=w305, y=1) -> (x+y=w303:i32)
          }
          frame "U04" {
            n190 = Add(x=w308, y=1) -> (x+y=w306:i32)
          }
          frame "U05" {
            n191 = Add(x=w311, y=1) -> (x+y=w309:i32)
          }
          frame "U06" {
            n192 = Add(x=w314, y=1) -> (x+y=w312:i32)
          }
          frame "U07" {
            n193 = Add(x=w317, y=1) -> (x+y=w315:i32)
          }
          frame "U08" {
            n194 = Add(x=w320, y=1) -> (x+y=w318:i32)
          }
          frame "U09" {
            n195 = Add(x=w323, y=1) -> (x+y=w321:i32)
          }
          frame "U10" {
            n196 = Add(x=w326, y=1) -> (x+y=w324:i32)
          }
        }
        n197 = flat-sequence {
          tunnel: w296 -> [w336]
          tunnel: [w334] -> w295
          tunnel: w293 -> [w332]
          tunnel: [w329] -> w292
          tunnel: [w328] -> w291
          tunnel: [w327] -> w290
          tunnel: w295 -> [w340]
          tunnel: w292 -> [w339]
          tunnel: w291 -> [w338]
          tunnel: w290 -> [w337]
          frame #0 {
            n198 = invoke on="インボークノード" class="LightColorMISDK" method="GetCalibData"(reference=w336, "calibrationCh"=w332, "comPort"=0) -> ("GetCalibData"=w333:refnum<k24>, "measurementDataList"=w334:refnum<k24>, "correctDataList"=w327:refnum<k24>, "colorValueCalibrationData"=w328:refnum<k24>)  [unwired: 5 in, 4 out]
            n199 = property on="プロパティノード" class="ReturnMessage"(reference=w333) -> ("errorCode"=w331:i32)  [unwired: 1 in, 2 out]
            "ErrorCode" <- w331
            n200 = Equal?(x=w331, y=0) -> (x = y?=w329:bool)
          }
          frame #1 {
            n201 = case shown="TRUE" w339 {
              tunnel: w340 -> [_ w359]
              tunnel: w338 -> [_ w358]
              tunnel: w337 -> [_ w343]
              frame False {
                n202 = property on="ID" class="Str"("Value"="") -> ()  [unwired: 2 in, 2 out]
              }
              frame True {
                n203 = control-ref of="After_B"() -> (w353:refnum<vi>)
                n204 = control-ref of="After_G"() -> (w351:refnum<vi>)
                n205 = control-ref of="After_W"() -> (w344:refnum<vi>)
                n206 = control-ref of="After_R"() -> (w349:refnum<vi>)
                n207 = control-ref of="Before_G"() -> (w350:refnum<vi>)
                n208 = control-ref of="Before_G 2"() -> (w347:refnum<vi>)
                n209 = control-ref of="Before_B 2"() -> (w345:refnum<vi>)
                n210 = control-ref of="Before_W 2"() -> (w354:refnum<vi>)
                n211 = control-ref of="Before_R 2"() -> (w348:refnum<vi>)
                n212 = control-ref of="Before_W"() -> (w355:refnum<vi>)
                n213 = property on="プロパティノード" class="UserCalibData"(reference=w358) -> ("CalibType"=w356:i32, "Id"=w342:string)  [unwired: 1 in, 2 out]
                n214 = control-ref of="Before_R"() -> (w346:refnum<vi>)
                n215 = case shown="0, デフォルト" w356 {
                  tunnel: [1 3 4] -> w357
                  frame 0, Default {
                  }
                  frame 1 {
                  }
                  frame 2 {
                  }
                }
                n216 = control-ref of="Before_B"() -> (w352:refnum<vi>)
                n217 = property on="Type of Calibration" class="RadioBtnsControl （指定）"("Value"=w356) -> ()  [unwired: 2 in, 2 out]
                n218 = property on="ID" class="Str"("Value"=w342) -> ()  [unwired: 2 in, 2 out]
                n219 = call "LC-MISDK_UserCalibration_TypeofCalib.vi"("Cluster入力"=w355, "Bool refnum 3"=w347, "Clust refnum 4"=w349, "Bool refnum 2"=w348, "Clust refnum 5"=w350, "Clust refnum 3"=w346, "Clust refnum 6"=w351, "Bool refnum 4"=w345, "Clust refnum 7"=w352, "Clust refnum入力"=w344, "Clust refnum 8"=w353, "Type of Calibration"=w356, "Bool refnum"=w354) -> ()  [unwired: 7 in]
                n220 = for {
                  N: w357 -> [w381]
                  tunnel: w359 -> [w385]
                  tunnel: w343 -> [w376]
                  i -> [w374]
                  n221 = invoke on="インボークノード" class="List`1[[Konicaminolta.Measureme" method="get_Item"(reference=w376, "index"=w374) -> ("get_Item"=w373:refnum<k24>)  [unwired: 2 in, 3 out]
                  n222 = invoke on="インボークノード" class="List`1[[Konicaminolta.Measureme" method="get_Item"(reference=w385, "index"=w374) -> (error out=w383:errorcluster, "get_Item"=w384:refnum<k24>)  [unwired: 2 in, 2 out]
                  n223 = property on="プロパティノード" class="MeasurementData"(reference=w373) -> ("ColorSpaceValue"=w372:refnum<k24>)  [unwired: 1 in, 2 out]
                  n224 = property on="プロパティノード" class="MeasurementData"(reference=w384, error in=w383) -> (error out=w364:errorcluster, "ColorSpaceValue"=w382:refnum<k24>, "ColorModeId"=w375:i32)  [unwired: 1 out]
                  n225 = property on="Color Space" class="Enum （指定）"("Value"=w375) -> ()  [unwired: 2 in, 2 out]
                  n226 = case shown="1" w375 {
                    tunnel: ["y" "vd" "duv" "Z" "Pe"] -> w369
                    tunnel: ["x" "ud" "Tcp" "Y" "λd"] -> w370
                    tunnel: ["Lv" "Lv" "Lv" "X" "Lv"] -> w371
                    frame 0, Default {
                    }
                    frame 1 {
                    }
                    frame 2 {
                    }
                    frame 3 {
                    }
                    frame 4 {
                    }
                  }
                  n227 = invoke class="Dictionary`2[[System.String, ms" method="get_Item"(reference=w372, error in=w364, "key"=w371) -> ("get_Item"=w368:dbl)  [unwired: 1 in, 3 out]
                  n228 = invoke class="Dictionary`2[[System.String, ms" method="get_Item"(reference=w372, error in=w364, "key"=w369) -> (error out=→"error out":errorcluster, "get_Item"=w366:dbl)  [unwired: 1 in, 2 out]
                  n229 = invoke class="Dictionary`2[[System.String, ms" method="get_Item"(reference=w372, error in=w364, "key"=w370) -> ("get_Item"=w367:dbl)  [unwired: 1 in, 3 out]
                  n230 = invoke on="インボークノード" class="Dictionary`2[[System.String, ms" method="get_Item"(reference=w382, "key"=w369) -> ("get_Item"=w378:dbl)  [unwired: 2 in, 3 out]
                  n231 = invoke on="インボークノード" class="Dictionary`2[[System.String, ms" method="get_Item"(reference=w382, "key"=w371) -> ("get_Item"=w380:dbl)  [unwired: 2 in, 3 out]
                  n232 = invoke on="インボークノード" class="Dictionary`2[[System.String, ms" method="get_Item"(reference=w382, "key"=w370) -> ("get_Item"=w379:dbl)  [unwired: 2 in, 3 out]
                  n233 = Bundle("get_Item"=w368, "get_Item"=w367, "get_Item"=w366) -> (w365:T11)  [unwired: 1 in]
                  n234 = Bundle("get_Item"=w380, "get_Item"=w379, "get_Item"=w378) -> (w377:T11)  [unwired: 1 in]
                  n235 = case shown="1, デフォルト" w381 {
                    tunnel: w377 -> [w547 w550 w559]
                    tunnel: w374 -> [_ w549 w558]
                    tunnel: w365 -> [w546 w548 w557]
                    frame 1, Default {
                      n236 = property on="Before_W" class="Clust （指定）"("Value"=w547) -> ()  [unwired: 2 in, 2 out]
                      n237 = property on="After_W" class="Clust （指定）"("Value"=w546) -> ()  [unwired: 2 in, 2 out]
                    }
                    frame 3 {
                      n238 = case shown="1" w549 {
                        tunnel: w550 -> [w552 w554 w556]
                        tunnel: w548 -> [w551 w553 w555]
                        frame 0, Default {
                          n239 = property on="Before_R" class="Clust （指定）"("Value"=w552) -> ()  [unwired: 2 in, 2 out]
                          n240 = property on="After_R" class="Clust （指定）"("Value"=w551) -> ()  [unwired: 2 in, 2 out]
                        }
                        frame 1 {
                          n241 = property on="Before_G" class="Clust （指定）"("Value"=w554) -> ()  [unwired: 2 in, 2 out]
                          n242 = property on="After_G" class="Clust （指定）"("Value"=w553) -> ()  [unwired: 2 in, 2 out]
                        }
                        frame 2 {
                          n243 = property on="Before_B" class="Clust （指定）"("Value"=w556) -> ()  [unwired: 2 in, 2 out]
                          n244 = property on="After_B" class="Clust （指定）"("Value"=w555) -> ()  [unwired: 2 in, 2 out]
                        }
                      }
                    }
                    frame 4 {
                      n245 = case shown="0, デフォルト" w558 {
                        tunnel: w559 -> [w561 w563 w565 w567]
                        tunnel: w557 -> [w560 w562 w564 w566]
                        frame 0, Default {
                          n246 = property on="Before_W" class="Clust （指定）"("Value"=w561) -> ()  [unwired: 2 in, 2 out]
                          n247 = property on="After_W" class="Clust （指定）"("Value"=w560) -> ()  [unwired: 2 in, 2 out]
                        }
                        frame 1 {
                          n248 = property on="Before_R" class="Clust （指定）"("Value"=w563) -> ()  [unwired: 2 in, 2 out]
                          n249 = property on="After_R" class="Clust （指定）"("Value"=w562) -> ()  [unwired: 2 in, 2 out]
                        }
                        frame 2 {
                          n250 = property on="Before_G" class="Clust （指定）"("Value"=w565) -> ()  [unwired: 2 in, 2 out]
                          n251 = property on="After_G" class="Clust （指定）"("Value"=w564) -> ()  [unwired: 2 in, 2 out]
                        }
                        frame 3 {
                          n252 = property on="Before_B" class="Clust （指定）"("Value"=w567) -> ()  [unwired: 2 in, 2 out]
                          n253 = property on="After_B" class="Clust （指定）"("Value"=w566) -> ()  [unwired: 2 in, 2 out]
                        }
                      }
                    }
                  }
                  n254 = case shown="1" w375 {
                    frame 0, Default {
                      w389 = refnum<vi> refnum  # テキスト
                      w394 = refnum<vi> refnum  # テキスト
                      w397 = refnum<vi> refnum  # テキスト
                      w404 = refnum<vi> refnum  # テキスト
                      w409 = refnum<vi> refnum  # テキスト
                      w414 = refnum<vi> refnum  # テキスト
                      n255 = property class="VI"() -> ("Panel"=w417:refnum<vi>)  [unwired: 2 in, 2 out]
                      n256 = property class="Pnl"(reference=w417) -> ("Decos[]"=w386:refnum<vi>[])  [unwired: 1 in, 2 out]
                      n257 = Index Array(array=w386, index=2) -> (element=w416:refnum<vi>)
                      n258 = Index Array(array=w386, index=17) -> (element=w399:refnum<vi>)
                      n259 = Index Array(array=w386, index=0) -> (element=w406:refnum<vi>)
                      n260 = Index Array(array=w386, index=1) -> (element=w411:refnum<vi>)
                      n261 = Index Array(array=w386, index=15) -> (element=w391:refnum<vi>)
                      n262 = Index Array(array=w386, index=16) -> (element=w396:refnum<vi>)
                      n263 = To More Specific Class(target class=w414, reference=w416) -> (specific class reference=w415:refnum<vi>)  [unwired: 1 in, 1 out]
                      n264 = To More Specific Class(target class=w397, reference=w399) -> (specific class reference=w401:refnum<vi>)  [unwired: 1 in, 1 out]
                      n265 = To More Specific Class(target class=w404, reference=w406) -> (specific class reference=w405:refnum<vi>)  [unwired: 1 in, 1 out]
                      n266 = To More Specific Class(target class=w409, reference=w411) -> (specific class reference=w410:refnum<vi>)  [unwired: 1 in, 1 out]
                      n267 = To More Specific Class(target class=w389, reference=w391) -> (specific class reference=w390:refnum<vi>)  [unwired: 1 in, 1 out]
                      n268 = To More Specific Class(target class=w394, reference=w396) -> (specific class reference=w395:refnum<vi>)  [unwired: 1 in, 1 out]
                      n269 = property class="Txt"(reference=w415, "Text"="Lv") -> ()  [unwired: 1 in, 2 out]
                      n270 = property class="Txt"(reference=w401, "Text"="Lv") -> ()  [unwired: 1 in, 2 out]
                      n271 = property class="Txt"(reference=w405, "Text"="y") -> ()  [unwired: 1 in, 2 out]
                      n272 = property class="Txt"(reference=w410, "Text"="x") -> ()  [unwired: 1 in, 2 out]
                      n273 = property class="Txt"(reference=w390, "Text"="y") -> ()  [unwired: 1 in, 2 out]
                      n274 = property class="Txt"(reference=w395, "Text"="x") -> ()  [unwired: 1 in, 2 out]
                    }
                    frame 1 {
                      w421 = refnum<vi> refnum  # テキスト
                      w426 = refnum<vi> refnum  # テキスト
                      w429 = refnum<vi> refnum  # テキスト
                      w436 = refnum<vi> refnum  # テキスト
                      w441 = refnum<vi> refnum  # テキスト
                      w446 = refnum<vi> refnum  # テキスト
                      n275 = property class="VI"() -> ("Panel"=w449:refnum<vi>)  [unwired: 2 in, 2 out]
                      n276 = property class="Pnl"(reference=w449) -> ("Decos[]"=w418:refnum<vi>[])  [unwired: 1 in, 2 out]
                      n277 = Index Array(array=w418, index=2) -> (element=w448:refnum<vi>)
                      n278 = Index Array(array=w418, index=17) -> (element=w431:refnum<vi>)
                      n279 = Index Array(array=w418, index=0) -> (element=w438:refnum<vi>)
                      n280 = Index Array(array=w418, index=1) -> (element=w443:refnum<vi>)
                      n281 = Index Array(array=w418, index=15) -> (element=w423:refnum<vi>)
                      n282 = Index Array(array=w418, index=16) -> (element=w428:refnum<vi>)
                      n283 = To More Specific Class(target class=w446, reference=w448) -> (specific class reference=w447:refnum<vi>)  [unwired: 1 in, 1 out]
                      n284 = To More Specific Class(target class=w429, reference=w431) -> (specific class reference=w433:refnum<vi>)  [unwired: 1 in, 1 out]
                      n285 = To More Specific Class(target class=w436, reference=w438) -> (specific class reference=w437:refnum<vi>)  [unwired: 1 in, 1 out]
                      n286 = To More Specific Class(target class=w441, reference=w443) -> (specific class reference=w442:refnum<vi>)  [unwired: 1 in, 1 out]
                      n287 = To More Specific Class(target class=w421, reference=w423) -> (specific class reference=w422:refnum<vi>)  [unwired: 1 in, 1 out]
                      n288 = To More Specific Class(target class=w426, reference=w428) -> (specific class reference=w427:refnum<vi>)  [unwired: 1 in, 1 out]
                      n289 = property class="Txt"(reference=w447, "Text"="Lv") -> ()  [unwired: 1 in, 2 out]
                      n290 = property class="Txt"(reference=w433, "Text"="Lv") -> ()  [unwired: 1 in, 2 out]
                      n291 = property class="Txt"(reference=w437, "Text"="v") -> ()  [unwired: 1 in, 2 out]
                      n292 = property class="Txt"(reference=w442, "Text"="u") -> ()  [unwired: 1 in, 2 out]
                      n293 = property class="Txt"(reference=w422, "Text"="v") -> ()  [unwired: 1 in, 2 out]
                      n294 = property class="Txt"(reference=w427, "Text"="u") -> ()  [unwired: 1 in, 2 out]
                    }
                    frame 2 {
                      w453 = refnum<vi> refnum  # テキスト
                      w458 = refnum<vi> refnum  # テキスト
                      w461 = refnum<vi> refnum  # テキスト
                      w468 = refnum<vi> refnum  # テキスト
                      w473 = refnum<vi> refnum  # テキスト
                      w478 = refnum<vi> refnum  # テキスト
                      n295 = property class="VI"() -> ("Panel"=w481:refnum<vi>)  [unwired: 2 in, 2 out]
                      n296 = property class="Pnl"(reference=w481) -> ("Decos[]"=w450:refnum<vi>[])  [unwired: 1 in, 2 out]
                      n297 = Index Array(array=w450, index=2) -> (element=w480:refnum<vi>)
                      n298 = Index Array(array=w450, index=17) -> (element=w463:refnum<vi>)
                      n299 = Index Array(array=w450, index=0) -> (element=w470:refnum<vi>)
                      n300 = Index Array(array=w450, index=1) -> (element=w475:refnum<vi>)
                      n301 = Index Array(array=w450, index=15) -> (element=w455:refnum<vi>)
                      n302 = Index Array(array=w450, index=16) -> (element=w460:refnum<vi>)
                      n303 = To More Specific Class(target class=w478, reference=w480) -> (specific class reference=w479:refnum<vi>)  [unwired: 1 in, 1 out]
                      n304 = To More Specific Class(target class=w461, reference=w463) -> (specific class reference=w465:refnum<vi>)  [unwired: 1 in, 1 out]
                      n305 = To More Specific Class(target class=w468, reference=w470) -> (specific class reference=w469:refnum<vi>)  [unwired: 1 in, 1 out]
                      n306 = To More Specific Class(target class=w473, reference=w475) -> (specific class reference=w474:refnum<vi>)  [unwired: 1 in, 1 out]
                      n307 = To More Specific Class(target class=w453, reference=w455) -> (specific class reference=w454:refnum<vi>)  [unwired: 1 in, 1 out]
                      n308 = To More Specific Class(target class=w458, reference=w460) -> (specific class reference=w459:refnum<vi>)  [unwired: 1 in, 1 out]
                      n309 = property class="Txt"(reference=w479, "Text"="Lv") -> ()  [unwired: 1 in, 2 out]
                      n310 = property class="Txt"(reference=w465, "Text"="Lv") -> ()  [unwired: 1 in, 2 out]
                      n311 = property class="Txt"(reference=w469, "Text"="duv") -> ()  [unwired: 1 in, 2 out]
                      n312 = property class="Txt"(reference=w474, "Text"="Tcp") -> ()  [unwired: 1 in, 2 out]
                      n313 = property class="Txt"(reference=w454, "Text"="duv") -> ()  [unwired: 1 in, 2 out]
                      n314 = property class="Txt"(reference=w459, "Text"="Tcp") -> ()  [unwired: 1 in, 2 out]
                    }
                    frame 3 {
                      w485 = refnum<vi> refnum  # テキスト
                      w490 = refnum<vi> refnum  # テキスト
                      w493 = refnum<vi> refnum  # テキスト
                      w500 = refnum<vi> refnum  # テキスト
                      w505 = refnum<vi> refnum  # テキスト
                      w510 = refnum<vi> refnum  # テキスト
                      n315 = property class="VI"() -> ("Panel"=w513:refnum<vi>)  [unwired: 2 in, 2 out]
                      n316 = property class="Pnl"(reference=w513) -> ("Decos[]"=w482:refnum<vi>[])  [unwired: 1 in, 2 out]
                      n317 = Index Array(array=w482, index=2) -> (element=w512:refnum<vi>)
                      n318 = Index Array(array=w482, index=17) -> (element=w495:refnum<vi>)
                      n319 = Index Array(array=w482, index=0) -> (element=w502:refnum<vi>)
                      n320 = Index Array(array=w482, index=1) -> (element=w507:refnum<vi>)
                      n321 = Index Array(array=w482, index=15) -> (element=w487:refnum<vi>)
                      n322 = Index Array(array=w482, index=16) -> (element=w492:refnum<vi>)
                      n323 = To More Specific Class(target class=w510, reference=w512) -> (specific class reference=w511:refnum<vi>)  [unwired: 1 in, 1 out]
                      n324 = To More Specific Class(target class=w493, reference=w495) -> (specific class reference=w497:refnum<vi>)  [unwired: 1 in, 1 out]
                      n325 = To More Specific Class(target class=w500, reference=w502) -> (specific class reference=w501:refnum<vi>)  [unwired: 1 in, 1 out]
                      n326 = To More Specific Class(target class=w505, reference=w507) -> (specific class reference=w506:refnum<vi>)  [unwired: 1 in, 1 out]
                      n327 = To More Specific Class(target class=w485, reference=w487) -> (specific class reference=w486:refnum<vi>)  [unwired: 1 in, 1 out]
                      n328 = To More Specific Class(target class=w490, reference=w492) -> (specific class reference=w491:refnum<vi>)  [unwired: 1 in, 1 out]
                      n329 = property class="Txt"(reference=w511, "Text"="X") -> ()  [unwired: 1 in, 2 out]
                      n330 = property class="Txt"(reference=w497, "Text"="X") -> ()  [unwired: 1 in, 2 out]
                      n331 = property class="Txt"(reference=w501, "Text"="Z") -> ()  [unwired: 1 in, 2 out]
                      n332 = property class="Txt"(reference=w506, "Text"="Y") -> ()  [unwired: 1 in, 2 out]
                      n333 = property class="Txt"(reference=w486, "Text"="Z") -> ()  [unwired: 1 in, 2 out]
                      n334 = property class="Txt"(reference=w491, "Text"="Y") -> ()  [unwired: 1 in, 2 out]
                    }
                    frame 4 {
                      w517 = refnum<vi> refnum  # テキスト
                      w522 = refnum<vi> refnum  # テキスト
                      w525 = refnum<vi> refnum  # テキスト
                      w532 = refnum<vi> refnum  # テキスト
                      w537 = refnum<vi> refnum  # テキスト
                      w542 = refnum<vi> refnum  # テキスト
                      n335 = property class="VI"() -> ("Panel"=w545:refnum<vi>)  [unwired: 2 in, 2 out]
                      n336 = property class="Pnl"(reference=w545) -> ("Decos[]"=w514:refnum<vi>[])  [unwired: 1 in, 2 out]
                      n337 = Index Array(array=w514, index=2) -> (element=w544:refnum<vi>)
                      n338 = Index Array(array=w514, index=17) -> (element=w527:refnum<vi>)
                      n339 = Index Array(array=w514, index=0) -> (element=w534:refnum<vi>)
                      n340 = Index Array(array=w514, index=1) -> (element=w539:refnum<vi>)
                      n341 = Index Array(array=w514, index=15) -> (element=w519:refnum<vi>)
                      n342 = Index Array(array=w514, index=16) -> (element=w524:refnum<vi>)
                      n343 = To More Specific Class(target class=w542, reference=w544) -> (specific class reference=w543:refnum<vi>)  [unwired: 1 in, 1 out]
                      n344 = To More Specific Class(target class=w525, reference=w527) -> (specific class reference=w529:refnum<vi>)  [unwired: 1 in, 1 out]
                      n345 = To More Specific Class(target class=w532, reference=w534) -> (specific class reference=w533:refnum<vi>)  [unwired: 1 in, 1 out]
                      n346 = To More Specific Class(target class=w537, reference=w539) -> (specific class reference=w538:refnum<vi>)  [unwired: 1 in, 1 out]
                      n347 = To More Specific Class(target class=w517, reference=w519) -> (specific class reference=w518:refnum<vi>)  [unwired: 1 in, 1 out]
                      n348 = To More Specific Class(target class=w522, reference=w524) -> (specific class reference=w523:refnum<vi>)  [unwired: 1 in, 1 out]
                      n349 = property class="Txt"(reference=w543, "Text"="Lv") -> ()  [unwired: 1 in, 2 out]
                      n350 = property class="Txt"(reference=w529, "Text"="Lv") -> ()  [unwired: 1 in, 2 out]
                      n351 = property class="Txt"(reference=w533, "Text"="Pe") -> ()  [unwired: 1 in, 2 out]
                      n352 = property class="Txt"(reference=w538, "Text"="λd") -> ()  [unwired: 1 in, 2 out]
                      n353 = property class="Txt"(reference=w518, "Text"="Pe") -> ()  [unwired: 1 in, 2 out]
                      n354 = property class="Txt"(reference=w523, "Text"="λd") -> ()  [unwired: 1 in, 2 out]
                    }
                  }
                }
              }
            }
          }
        }
      }
    }
  }
